vi "Write Picture.vi"(8 "error in (no error)":errorcluster, 10 "Picture":fxp<+,3,3>[](array[numeric]), 11 "RT_Sprite in":refnum<class "RT_Sprite.lvclass">) -> (0 "error out":errorcluster, 3 "RT_Sprite out":refnum<class "RT_Sprite.lvclass">)   [LabVIEW 2019, in "RT_Game.lvlib" / "RT_Sprite.lvclass"]
uses:
  RT_Sprite.lvclass
  RT_Sprite.lvclass/RT_Sprite.ctl
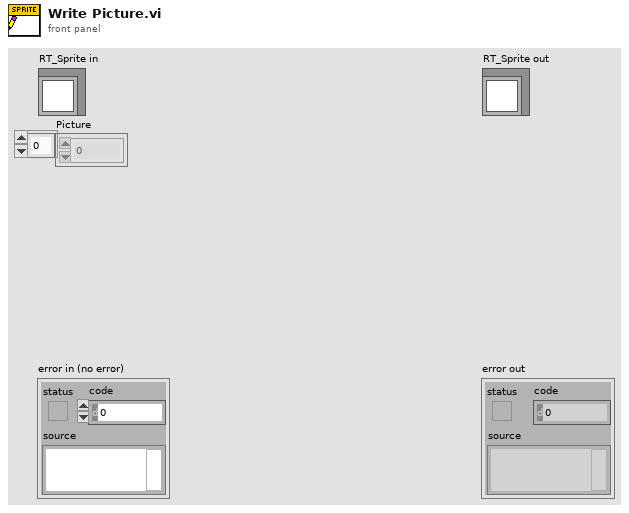
[diagram p1: front panel]
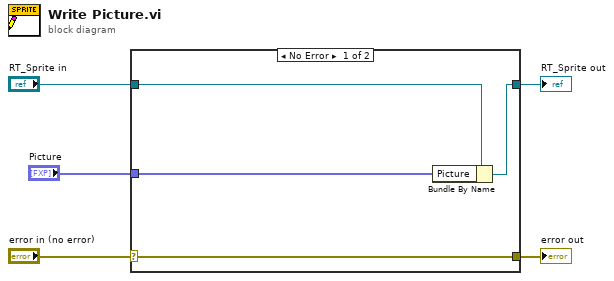
[diagram p0: block diagram]
diagram:
  n1 = case shown="No Error" "error in (no error)" {
    selector: "error in (no error)" -> [w9 w10]
    tunnel: [w9 w10] -> w4
    tunnel: [w7 w11] -> w2
    tunnel: "RT_Sprite in" -> [w8 w11]
    tunnel: "Picture" -> [w6 _]
    frame No Error {
      n2 = Bundle By Name(cluster=w8, "Picture"=w6) -> (w7:refnum<class "RT_Sprite.lvclass">)
    }
    frame Error {
    }
  }
  "error out" <- w4
  "RT_Sprite out" <- w2
